vi "Feeding.vi"(8 "error In":errorcluster) -> (0 "error out":errorcluster)   [LabVIEW 2017]
uses:
  Controls/LOADING_DISPLAY.ctl
  <vilib>/Utility/error.llb/DialogType.ctl
  Controls/Feed_Cyc_Data.ctl
  Controls/QUEUE_STATES.ctl
  Controls/Feed_St.ctl
  <vilib>/Utility/file.llb/Read Delimited Spreadsheet (string).vi
  <vilib>/Instr/_visa.llb/VISA Configure Serial Port (Instr).vi
panel:
  out "logical AND":bool
  out "element":u16
  out "Boolean array":bool[](array[boolean])
  out "output cluster 2":cluster{"RECIPE INDEX":i32, "COMBI BIN":i32}
  in  "Close _Door":bool
  out "raw scan code":string
  in  "BYPASS SCN":bool
  in  "String":string
  out "Scanner Comm":bool
  out "Stop scanner":bool
  out "CYCLE STATUS":string
  out "CURRENT PLAN":T1
  out "SCAN CODE:":string
  out "Selected Plan structure":string[][](table)
  out "Plan Selected:":string
  out "USER:-":string
  in  "Stop":bool
  out "DATE/TIME":string
  out "Screen Name":string
  # "DOOR NUMBER"
  # "SCANNED CODE"
  # "FEEDER STATUS"
  # "DOOR NUMBER"
  # "SCANNED CODE"
  # "FEEDER STATUS"
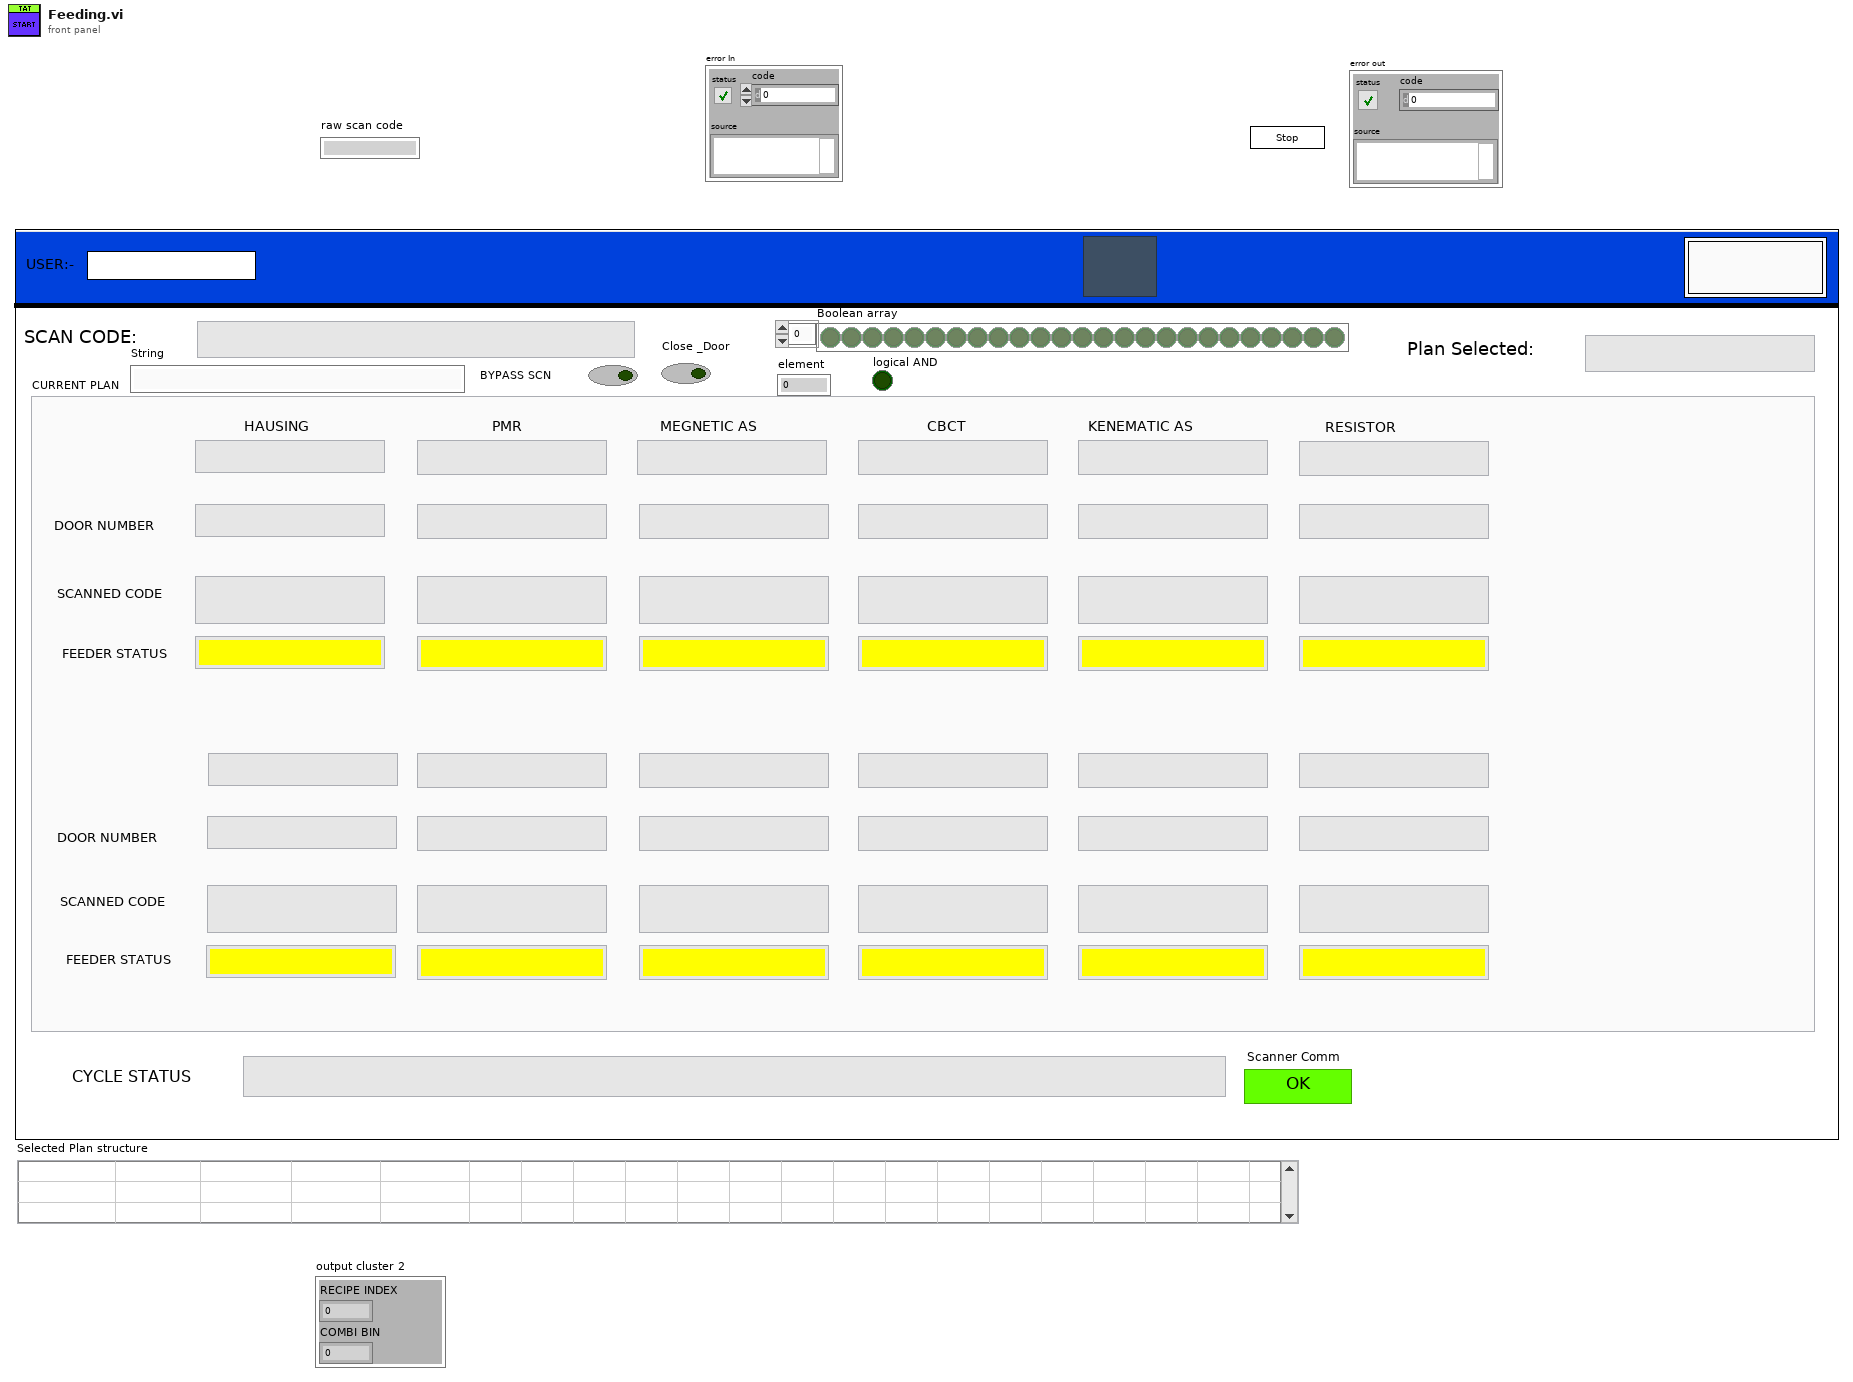
[diagram p1: front panel]
types:
  T1 = typedef "LOADING_DISPLAY.ctl" = cluster{"HAUSING":string, "PMR":string, "MEGNETIC AS":string, "CBCT":string, "KENEMATIC AS":string, "RESISTOR":string, "HAUSING DOOR":string, "PMR DOOR":string, "MAGNETIC AS DOOR":string, "CBCT DOOR":string, "KINEMATIC AS DOOR":string, "RESISTOR DOOR":string, "HAUSING SCAN QR":string, "PMR SCAN QR":string, "MAGNETIC SCAN QR":string, "CBCT SCAN QR":string, "KINEMATIC SCAN QR":string, "RESISTOR SCAN QR":string, "HAUSING FEED STATUS":string, "PMR FEED STATUS":string, "MAGNETIC AS FEEED STATUS":string, "CBCT FEED STATUS":string, "KINEMATIC AS FEED STATUS":string, "RESISTOR 1 FEED STATUS":string, "HAUSING 2":string, "PMR 2":string, "MEGNETIC AS 2":string, "CBCT 2":string, "KENEMATIC AS 2":string, "RESISTOR 2":string, "HAUSING DOOR 4":string, "PMR DOOR 4":string, "MAGNETIC AS DOOR 4":string, "CBCT DOOR 4":string, "KINEMATIC AS DOOR 4":string, "RESISTOR 1 DOOR 4":string, "HAUSING 2 SCAN QR":string, "PMR 2 SCAN QR":string, "MAGNETIC 2 SCAN QR":string, "CBCT 2 SCAN QR":string, "KINEMATIC 2 SCAN QR":string, "RESISTOR 2 SCAN QR":string, "HAUSING FEED STATUS 2":string, "PMR FEED STATUS 2":string, "MAGNETIC AS FEEED STATUS 2":string, "CBCT FEED STATUS 2":string, "KINEMATIC AS FEED STATUS 2":string, "RESISTOR 1 FEED STATUS 2":string}
  T2 = typedef "Feed_Cyc_Data.ctl" = cluster{"Cycle_Plan":path, "Plan_Data":string[][], "Scanned_Data":string[], "Scanned Chld Part":cluster{"Selected Door No":string, "child part code":string, "chld prt Row":i32, "Chld Prt Index":i32, "Scanned Data":string}, "feed Status Indi":refnum<vi>[], "Recipe Selected":cluster{"Bin/Box Mode":i32, "Selected Section":i32, "SELTED RECP & COMBI BIN":cluster{i32, i32}, "SELECTED RECIPE":string}}
  T3 = typedef "DialogType.ctl" = u16
  T4 = enum32{"invalid app kind", "Development System", "Run Time System", "Student Edition", "Embedded LabVIEW", "Evaluation", "Custom"}
  T5 = typedef "QUEUE_STATES.ctl" = enum16{"CREATE Q", "EN Q", "DE Q", "CLOSE Q"}
  T6 = cluster{"Printer IP":string, "PLC IP Address":string, "Scanner Com":refnum<visa-resource-name>}
  T7 = typedef "Feed_St.ctl" = enum16{"Int 2", "Cluster_update", "Read_Plan", "QR_Scanned", "Int", "SaveReport ", "Error_Handler", "Wait", "Close_Door", "Stop"}
  T8 = cluster{"Selected Door No":string, "child part code":string, "chld prt Row":i32, "Chld Prt Index":i32, "Scanned Data":string}
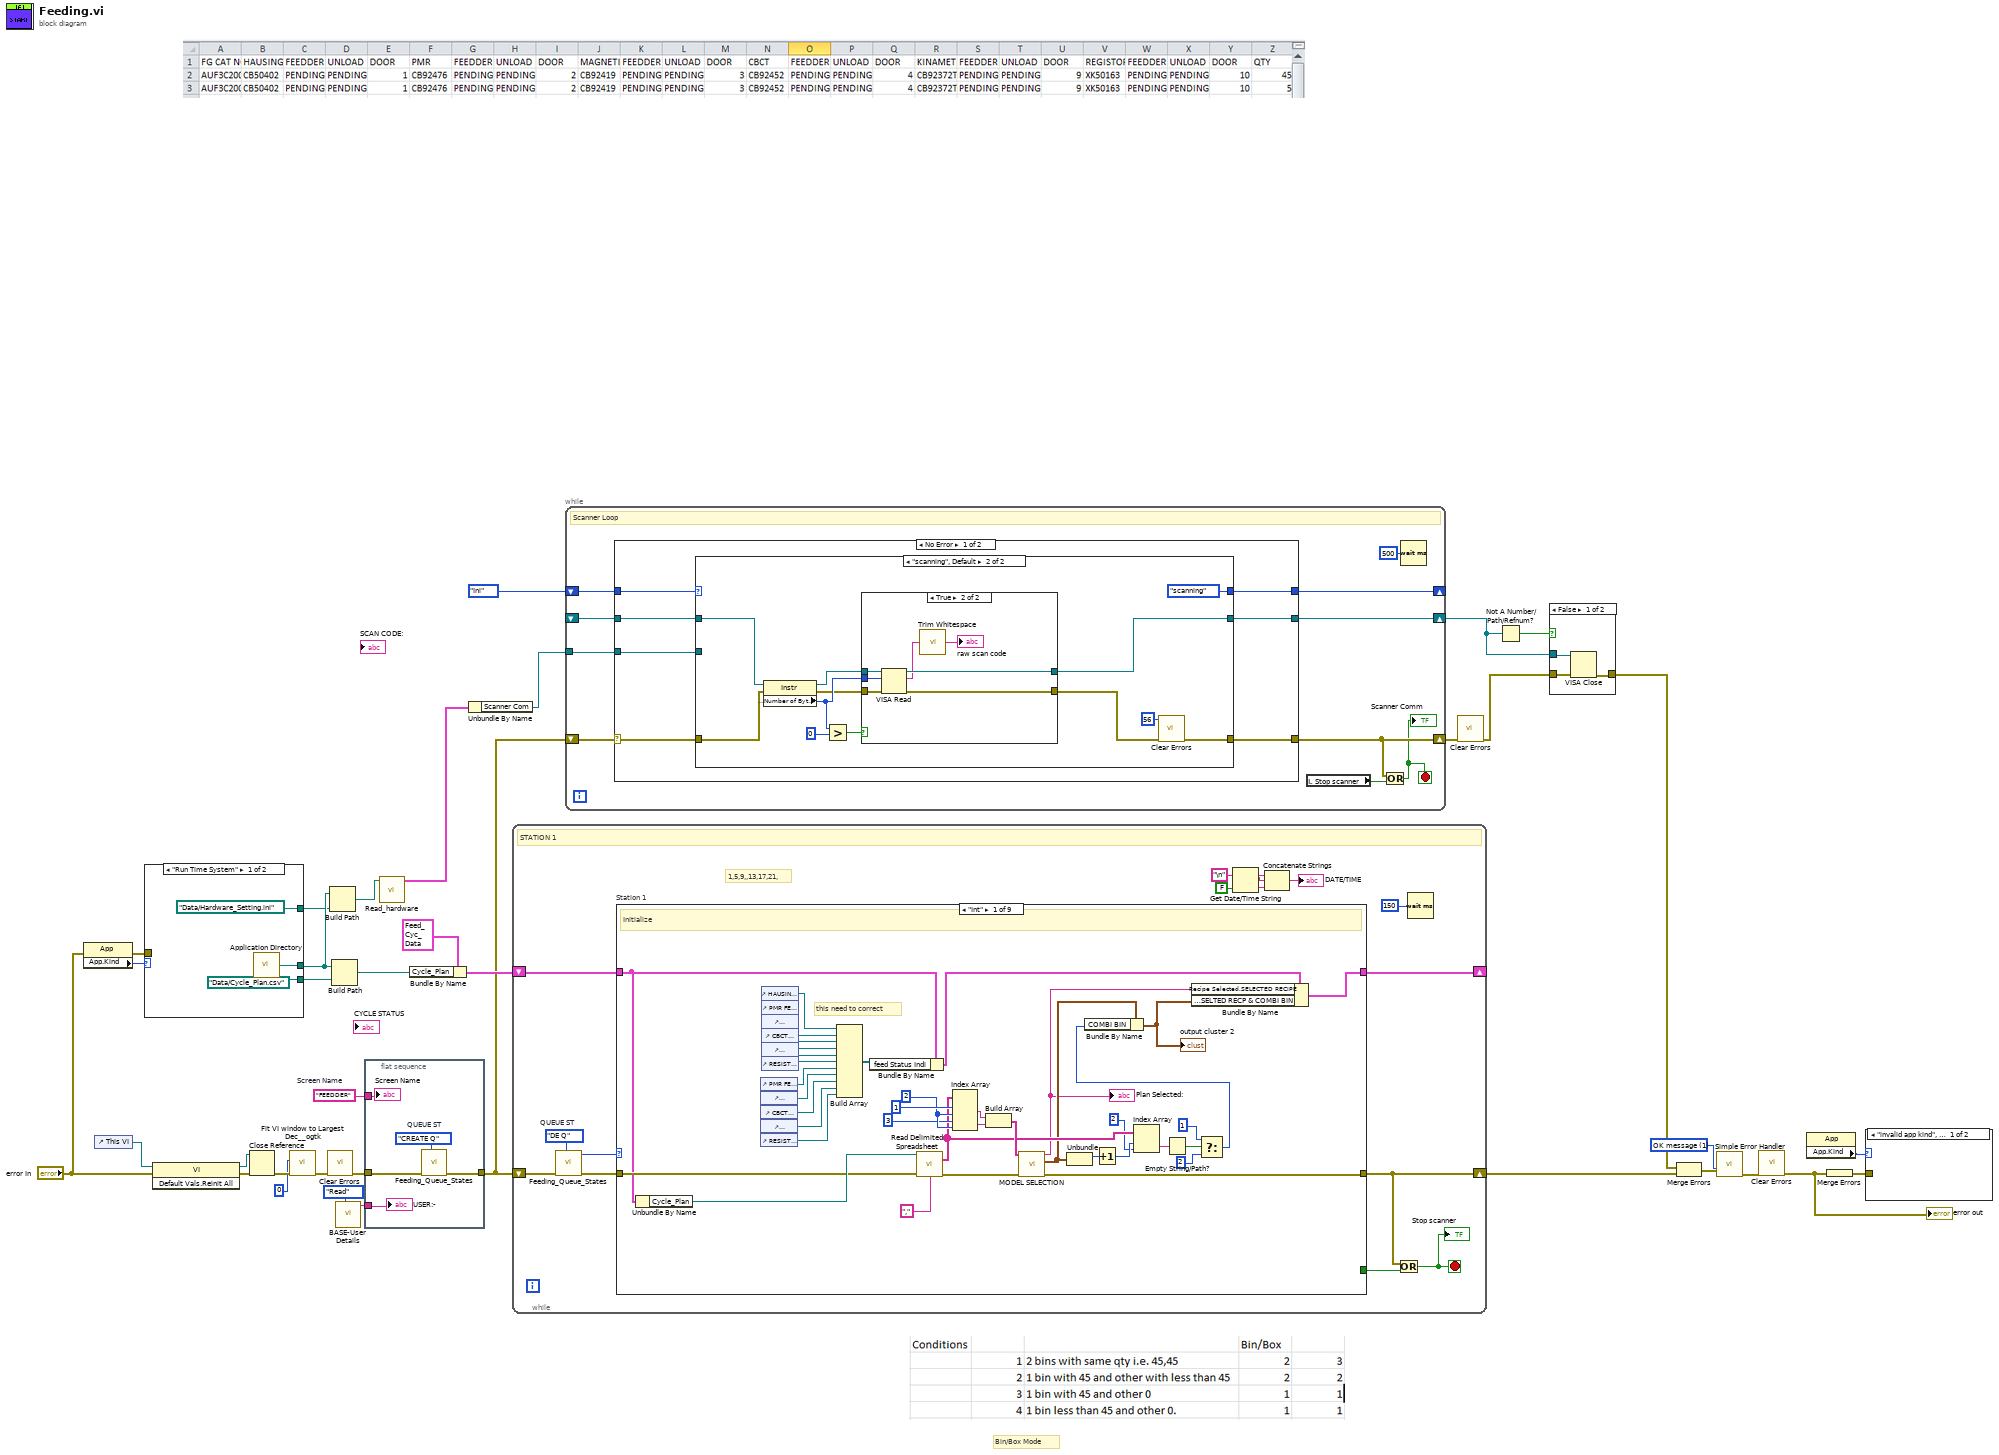
[diagram p0: block diagram]
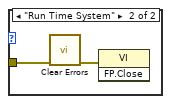
[diagram p2: hidden frame]
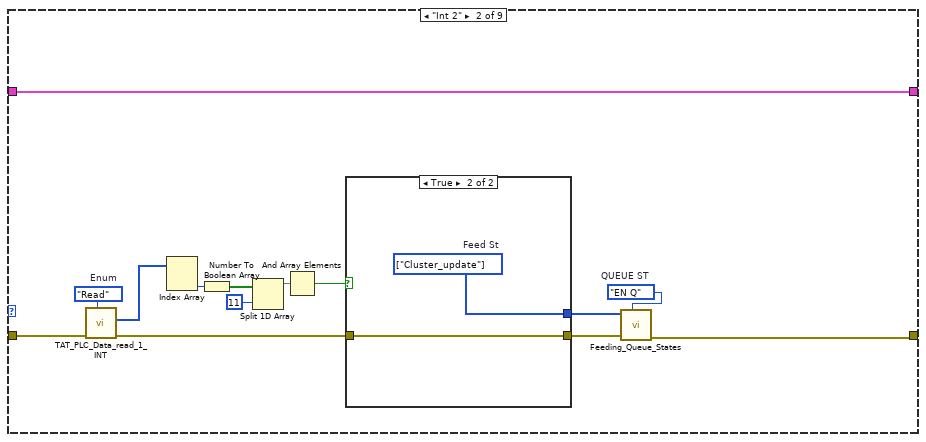
[diagram p3: hidden frame]
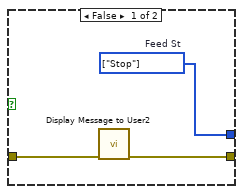
[diagram p4: hidden frame]
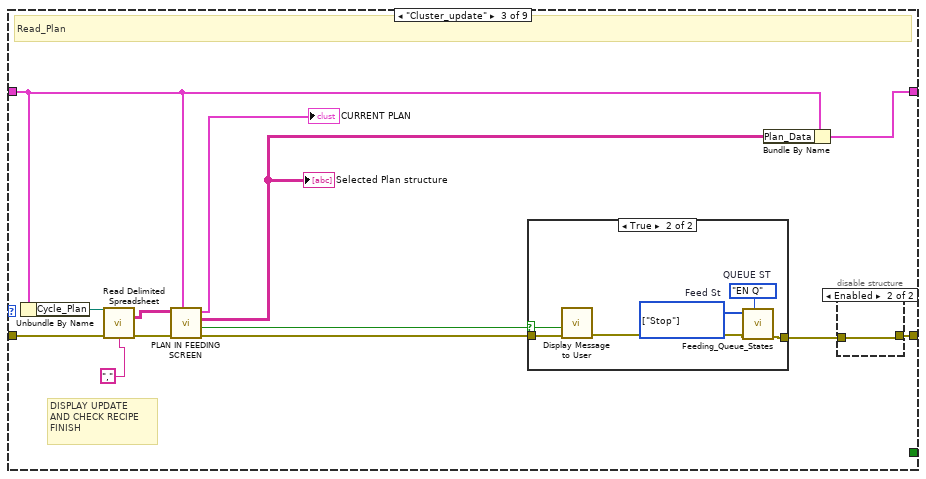
[diagram p5: hidden frame]
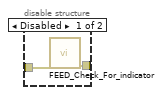
[diagram p6: hidden frame]
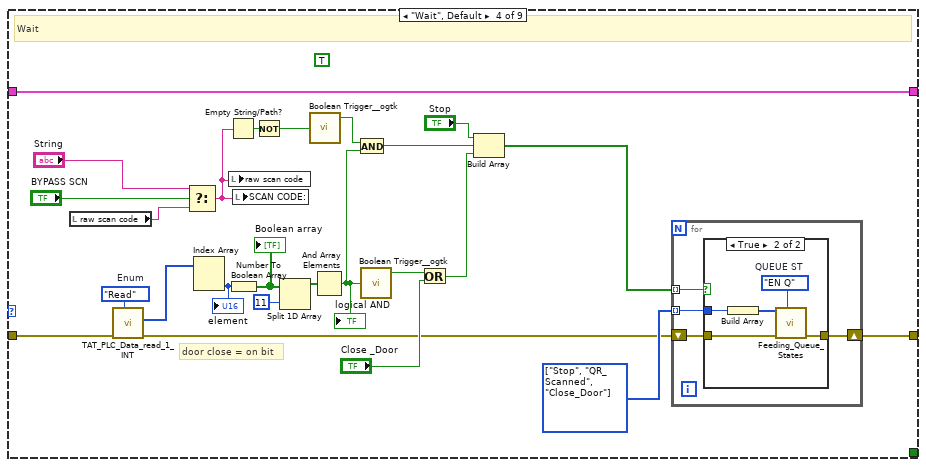
[diagram p8: hidden frame]
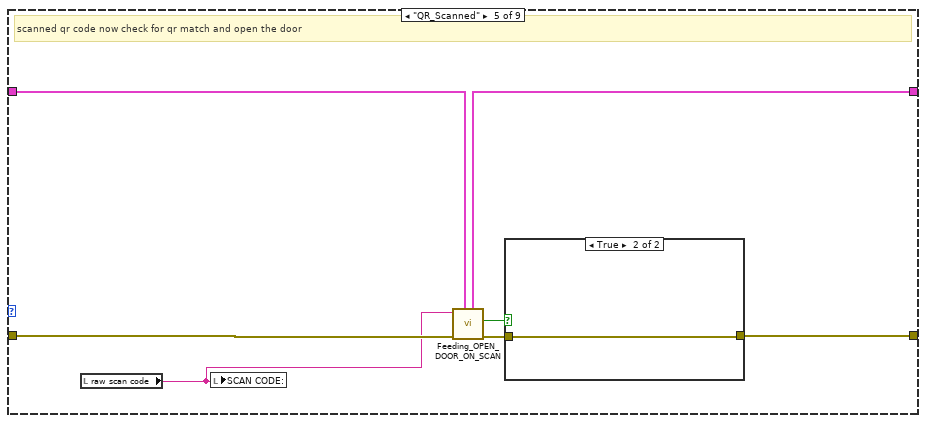
[diagram p10: hidden frame]
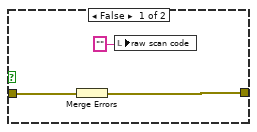
[diagram p11: hidden frame]
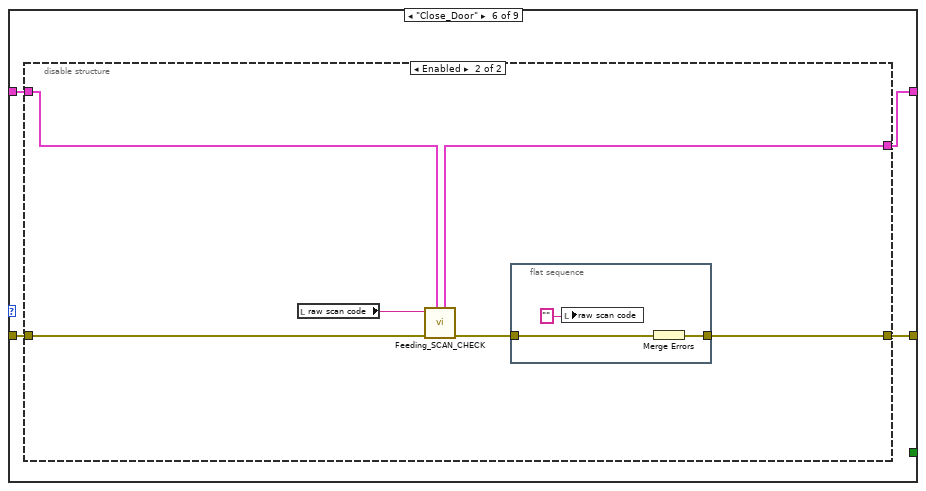
[diagram p12: hidden frame]
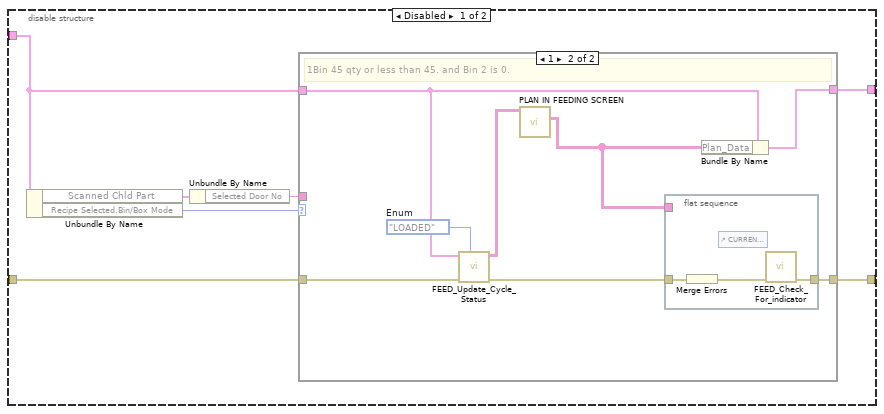
[diagram p13: hidden frame]
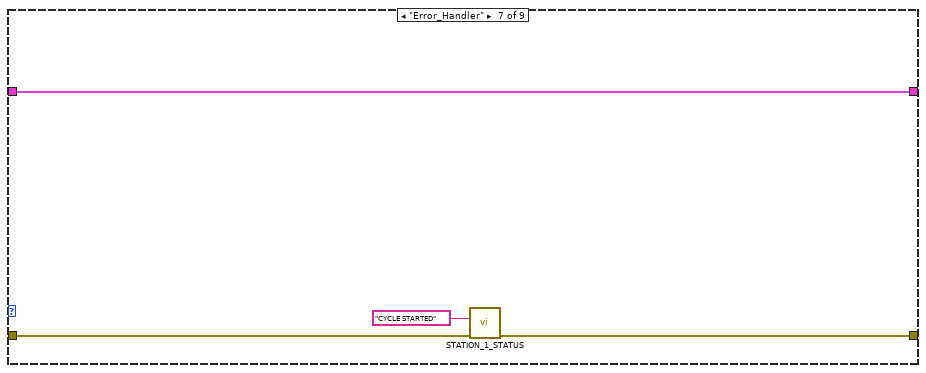
[diagram p15: hidden frame]
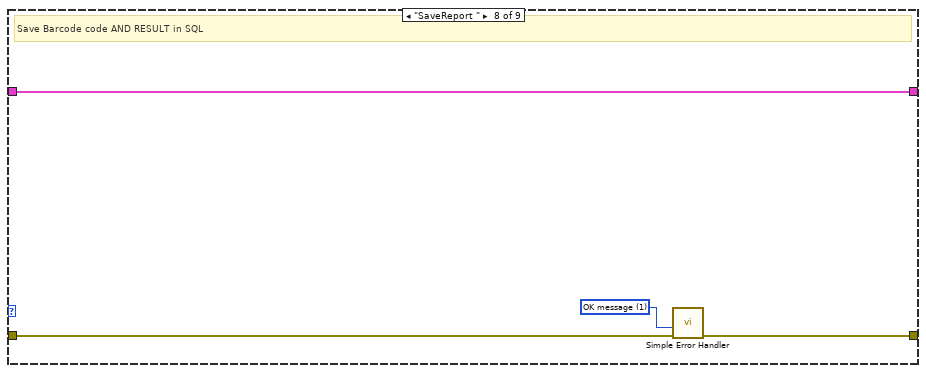
[diagram p16: hidden frame]
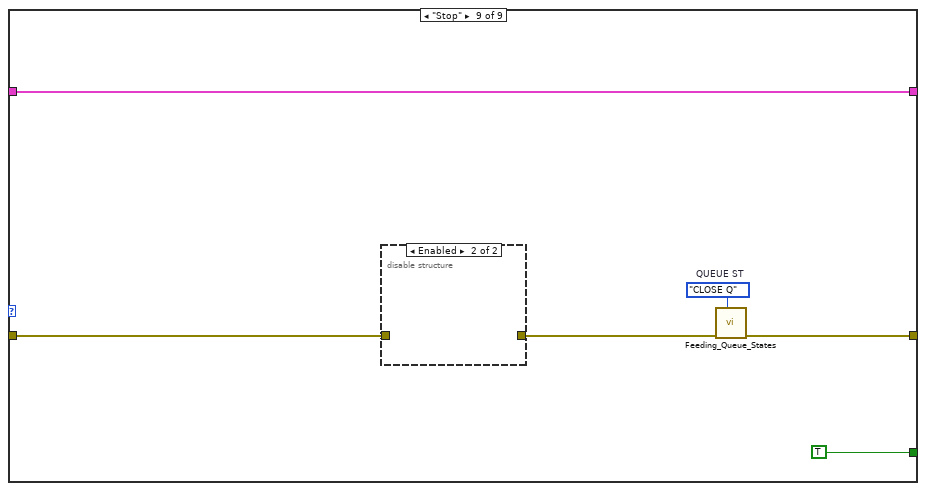
[diagram p17: hidden frame]
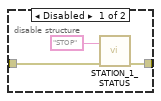
[diagram p18: hidden frame]
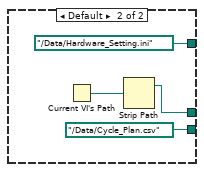
[diagram p19: hidden frame]
diagram:
  w17 = "FEEDDER"  # Screen Name
  w29 = T3 1 items=["no dialog", "OK message", "continue or stop message", "OK message + warnings", "continue/stop + warnings"] ("type of dialog (OK msg:1)")
  # "Bin/Box Mode"
  n1 = property class="App"(error in="error In") -> (error out=w25:errorcluster, "App.Kind"=w27:T4)  [unwired: 1 in, 1 out]
  n2 = control-ref of="This VI"() -> (w36:refnum<vi>)
  n3 = case shown="\"Run Time System\"" w27 {
    tunnel: [path "Data/Cycle_Plan.csv" ("path") path "../Data/Cycle_Plan.csv" ("path")] -> w26
    tunnel: [w37 w41] -> w6
    tunnel: w25 -> [_ _]
    tunnel: [path "Data/Hardware_Setting.ini" ("path") path "../Data/Hardware_Setting.ini" ("path")] -> w5
    frame "Run Time System" {
      n4 = call <vilib>:"Application Directory.vi"() -> ("Application Directory"=w37:path)
    }
    frame Default {
      n5 = Current VI's Path() -> (path=w42:path)
      n6 = Strip Path(path=w42) -> (stripped path=w41:path)  [unwired: 1 out]
    }
  }
  n7 = invoke class="VI" method="Default Vals.Reinit All"(reference=w36, error in="error In") -> (reference out=w34:refnum<vi>, error out=w35:errorcluster)  [unwired: 1 in, 1 out]
  n8 = Close Reference(reference=w34, error in (no error)=w35) -> (error out=w33:errorcluster)
  n9 = call <userlib>:"Fit VI window to Largest Dec__ogtk.vi"("error in (no error)"=w33, "border spacing (2 px)"=0) -> ("error out"=w23:errorcluster)  [unwired: 4 in, 1 out]
  n10 = call <vilib>:"Clear Errors.vi"("error in (no error)"=w23) -> ("error out"=w10:errorcluster)  [unwired: 5 in, 1 out]
  n11 = Build Path(base path=w6, name or relative path=w5) -> (appended path=w4:path)
  n12 = Build Path(base path=w6, name or relative path=w26) -> (appended path=w19:path)
  n13 = call "BASE-User Details.vi"("Enum"=enum16{"Read", "Write"}."Read") -> ("User Name Out"=w30:string)  [unwired: 9 in, 1 out]
  n14 = flat-sequence {
    tunnel: [w45] -> w11
    tunnel: w10 -> [w46]
    tunnel: w30 -> [w48]
    tunnel: w17 -> [w47]
    frame #0 {
      w44 = QUEUE_STATES."CREATE Q"  # QUEUE ST
      n15 = call "Feeding_Queue_States.vi"("QUEUE ST"=w44, "error in"=w46) -> ("error OUT"=w45:errorcluster)  [unwired: 8 in, 1 out]
      "USER:-" <- w48
      "Screen Name" <- w47
    }
  }
  n16 = call "Read_hardware.vi"("configuration file path"=w4) -> ("data"=w8:T6)  [unwired: 10 in]
  n17 = Bundle By Name(cluster=T2 {"Cycle_Plan"=path "", "Plan_Data"=[], "Scanned_Data"=[], "Scanned Chld Part"={"Selected Door No"="", "child part code"="", "chld prt Row"=0, "Chld Prt Index"=0, "Scanned Data"=""}, "feed Status Indi"=[], "Recipe Selected"={"Bin/Box Mode"=0, "Selected Section"=0, "SELTED RECP & COMBI BIN"={0, 0}, "SELECTED RECIPE"=""}}, "Cycle_Plan"=w19) -> (w18:T2)
  n18 = Unbundle By Name(w8) -> ("Scanner Com"=w7:refnum<visa-resource-name>)
  n19 = while {
    shift-right: [w55] -> _
    shift-left: w18 -> [w56]
    shift-right: [w53] -> w9
    shift-left: w11 -> [w52]
    stop <- w54 stop-if-true
    w50 = QUEUE_STATES."DE Q"  # QUEUE ST
    # "1,5,9,,13,17,21,"
    # "STATION 1"
    n20 = call "Feeding_Queue_States.vi"("QUEUE ST"=w50, "error in"=w52) -> ("error OUT"=w51:errorcluster, "Feed ST"=w49:T7)  [unwired: 8 in]
    n21 = case "Station 1" shown="\"Int\"" w49 {
      tunnel: [_ _ _ _ _ _ _ _ TRUE] -> w57
      tunnel: [w64 w104 w127 w165 w180 w192 w224 w229 w231] -> w53
      tunnel: w51 -> [w86 w108 w132 w154 w185 w193 w225 w228 w235]
      tunnel: w56 -> [w77 w115 w122 w168 w182 w191 w223 w227 w234]
      tunnel: [w78 w115 w126 w168 w181 w190 w223 w227 w234] -> w55
      frame "Int" {
        w83 = 2
        # "this need to correct"
        # "Initialize"
        n22 = Unbundle By Name(w77) -> ("Cycle_Plan"=w89:path)
        n23 = control-ref of="PMR FEED STATUS 2"() -> (w97:refnum<vi>)
        n24 = control-ref of="MAGNETIC AS FEEED STATUS 2"() -> (w98:refnum<vi>)
        n25 = control-ref of="CBCT FEED STATUS 2"() -> (w99:refnum<vi>)
        n26 = control-ref of="KINEMATIC AS FEED STATUS 2"() -> (w100:refnum<vi>)
        n27 = control-ref of="RESISTOR 1 FEED STATUS 2"() -> (w101:refnum<vi>)
        n28 = control-ref of="HAUSING FEED STATUS"() -> (w91:refnum<vi>)
        n29 = control-ref of="PMR FEED STATUS"() -> (w92:refnum<vi>)
        n30 = control-ref of="MAGNETIC AS FEEED STATUS"() -> (w93:refnum<vi>)
        n31 = control-ref of="CBCT FEED STATUS"() -> (w94:refnum<vi>)
        n32 = control-ref of="KINEMATIC AS FEED STATUS"() -> (w95:refnum<vi>)
        n33 = control-ref of="RESISTOR 1 FEED STATUS"() -> (w96:refnum<vi>)
        n34 = Build Array(w91, w92, w93, w94, w95, w96, w97, w98, w99, w100, w101) -> (w90:refnum<vi>[])
        n35 = Bundle By Name(cluster=w77, "feed Status Indi"=w90) -> (w79:T2)
        n36 = call-poly <vilib>:"Read Delimited Spreadsheet.vi"("file path (dialog if empty)"=w89, "error in (no error)"=w86, "delimiter (\\t)"=",") -> ("all rows"=w76:string[][], "error out"=w85:errorcluster)  [unwired: 7 in, 4 out]
        n37 = Index Array(array=w76, index (row) #1=1, index (col) #1=w83, index (row) #2=3, index (col) #2=w83) -> (element #1=w81:string, element #2=w80:string)
        n38 = Build Array(w81, w80) -> (w88:string[])
        n39 = call "MODEL SELECTION.vi"("error in (no error)"=w85, "Plan List"=w88) -> ("error out 2"=w64:errorcluster, "SELECTED RECIPE\nand COMBI OF BIN- INDEX"=w68:cluster{"RECIPE INDEX":i32, "COMBI BIN":i32}, "Plan Selected"=w65:string)  [unwired: 7 in]
        "Plan Selected:" <- w65
        n40 = Unbundle(w68) -> ("RECIPE INDEX"=w75:i32)  [unwired: 1 out]
        n41 = Increment(x=w75) -> (x+1=w74:i32)
        n42 = Index Array(array=w76, index (row)=w74, index (col)=2) -> (element=w72:string)
        n43 = Empty String/Path?(string/path=w72) -> (empty?=w71:bool)
        n44 = Select(t=1, s=w71, f=2) -> (s? t:f=w66:i32)
        n45 = Bundle By Name(cluster=w68, "COMBI BIN"=w66) -> (w67:cluster{"RECIPE INDEX":i32, "COMBI BIN":i32})
        "output cluster 2" <- w67
        n46 = Bundle By Name(cluster=w79, "Recipe Selected.SELECTED RECIPE"=w65, "Recipe Selected.SELTED RECP & COMBI BIN"=w67) -> (w78:T2)
      }
      frame "Int 2" {
        w106 = QUEUE_STATES."EN Q"  # QUEUE ST
        w114 = enum16{"Read", "Write"}."Read"  # Enum
        n47 = call "TAT_PLC_Data_read_1_INT.vi"("Enum"=w114, "error in (no error)"=w108) -> ("error out"=w107:errorcluster, "Array 2"=w113:u16[])  [unwired: 8 in]
        n48 = Index Array(array=w113) -> (element #2=w112:u16)  [unwired: 2 in, 1 out]
        n49 = Number To Boolean Array(number=w112) -> (Boolean array=w111:bool[])
        n50 = Split 1D Array(array=w111, index=11) -> (first subarray=w109:bool[])  [unwired: 1 out]
        n51 = And Array Elements(Boolean array=w109) -> (logical AND=w102:bool)
        n52 = case shown="True" w102 {
          tunnel: w107 -> [w117 w119]
          tunnel: [w116 w119] -> w103
          tunnel: [w118 w120] -> w105
          frame False {
            w118 = T7[] [enum."Stop"] items=["Int 2", "Cluster_update", "Read_Plan", "QR_Scanned", "Int", "SaveReport ", "Error_Handler", "Wait", "Close_Door", "Stop"]  # Feed St
            n53 = call "Display Message to User2"("error in (no error)"=w117) -> ("error out"=w116:errorcluster)  [unwired: 9 in, 1 out]
          }
          frame True {
            w120 = T7[] [enum."Cluster_update"] items=["Int 2", "Cluster_update", "Read_Plan", "QR_Scanned", "Int", "SaveReport ", "Error_Handler", "Wait", "Close_Door", "Stop"]  # Feed St
          }
        }
        n54 = call "Feeding_Queue_States.vi"("QUEUE ST"=w106, "error in"=w103, "Feed St"=w105) -> ("error OUT"=w104:errorcluster)  [unwired: 7 in, 1 out]
      }
      frame "Cluster_update" {
        # "DISPLAY UPDATE\nAND CHECK RECIPE\nFINISH"
        # "Read_Plan"
        n55 = Unbundle By Name(w122) -> ("Cycle_Plan"=w131:path)
        n56 = call-poly <vilib>:"Read Delimited Spreadsheet.vi"("file path (dialog if empty)"=w131, "error in (no error)"=w132, "delimiter (\\t)"=",") -> ("all rows"=w129:string[][], "error out"=w124:errorcluster)  [unwired: 7 in, 4 out]
        n57 = call "PLAN IN FEEDING SCREEN.vi"("LOOP DATA IN"=w122, "error IN"=w124, "PLAN In"=w129) -> ("error out"=w125:errorcluster, "NO EMPTY CMPLT?"=w121:bool, "PLAN Out"=w130:string[][], "CURRENT PLAN"=→"CURRENT PLAN":T1)  [unwired: 4 in]
        "Selected Plan structure" <- w130
        n58 = case shown="True" w121 {
          selector: w121 -> [_ w138]
          tunnel: w125 -> [w137 w140]
          tunnel: [w137 w142] -> w128
          frame False {
          }
          frame True {
            w141 = T7[] [enum."Stop"] items=["Int 2", "Cluster_update", "Read_Plan", "QR_Scanned", "Int", "SaveReport ", "Error_Handler", "Wait", "Close_Door", "Stop"]  # Feed St
            w143 = QUEUE_STATES."EN Q"  # QUEUE ST
            n59 = call "Display Message to User"("error in (no error)"=w140, "Enable"=w138) -> ("error out"=w139:errorcluster)  [unwired: 8 in, 1 out]
            n60 = call "Feeding_Queue_States.vi"("QUEUE ST"=w143, "error in"=w139, "Feed St"=w141) -> ("error OUT"=w142:errorcluster)  [unwired: 7 in, 1 out]
          }
        }
        n61 = Bundle By Name(cluster=w122, "Plan_Data"=w130) -> (w126:T2)
        n62 = disable-structure shown="Enabled" {
          disable-tunnel: w128 -> [w135 w136]
          disable-tunnel: [w134 w136] -> w127
          frame Disabled {
            n63 = call "FEED_Check_For_indicator.vi"("error in (no error)"=w135) -> ("error out"=w134:errorcluster)  [unwired: 10 in]
          }
          frame Enabled {
          }
        }
      }
      frame "Wait", Default {
        (unwired) TRUE
        w152 = enum16{"Read", "Write"}."Read"  # Enum
        w161 = T7[] [enum."Stop", enum."QR_Scanned", enum."Close_Door"] items=["Int 2", "Cluster_update", "Read_Plan", "QR_Scanned", "Int", "SaveReport ", "Error_Handler", "Wait", "Close_Door", "Stop"] ("Array")
        # "door close = on bit"
        # "Wait"
        n64 = local read "raw scan code"() -> (w160:string)
        n65 = call "TAT_PLC_Data_read_1_INT.vi"("Enum"=w152, "error in (no error)"=w154) -> ("error out"=w153:errorcluster, "Array 2"=w151:u16[])  [unwired: 8 in]
        n66 = Select(t="String", s="BYPASS SCN", f=w160) -> (s? t:f=w157:string)
        n67 = Index Array(array=w151) -> (element #2=w148:u16)  [unwired: 2 in, 1 out]
        "element" <- w148
        n68 = Empty String/Path?(string/path=w157) -> (empty?=w164:bool)
        n69 = local write "raw scan code"(w157) -> ()
        n70 = Number To Boolean Array(number=w148) -> (Boolean array=w147:bool[])
        "Boolean array" <- w147
        n71 = local write "SCAN CODE:"(w157) -> ()
        n72 = Not(x=w164) -> (.not. x?=w156:bool)
        n73 = Split 1D Array(array=w147, index=11) -> (first subarray=w145:bool[])  [unwired: 1 out]
        n74 = call <userlib>:"Boolean Trigger__ogtk.vi"("Boolean Input"=w156) -> ("Rising Edge"=w155:bool)  [unwired: 1 in, 1 out]
        n75 = And Array Elements(Boolean array=w145) -> (logical AND=w144:bool)
        "logical AND" <- w144
        n76 = And(x=w155, y=w144) -> (x .and. y?=w150:bool)
        n77 = call <userlib>:"Boolean Trigger__ogtk.vi"("Boolean Input"=w144) -> ("Rising Edge"=w149:bool)  [unwired: 1 in, 1 out]
        n78 = Or(x=w149, y="Close _Door") -> (x .or. y?=w158:bool)
        n79 = Build Array("Stop", w150, w158) -> (w162:bool[])
        n80 = for {
          shift-right: [w171] -> w165
          shift-left: w153 -> [w172]
          tunnel: w162 -> [w170] mode=indexing
          tunnel: w161 -> [w169] mode=indexing
          n81 = case shown="True" w170 {
            tunnel: w172 -> [w173 w177]
            tunnel: [w173 w176] -> w171
            tunnel: w169 -> [_ w175]
            frame False {
            }
            frame True {
              w178 = QUEUE_STATES."EN Q"  # QUEUE ST
              n82 = Build Array(w175) -> (w174:T7[])
              n83 = call "Feeding_Queue_States.vi"("QUEUE ST"=w178, "error in"=w177, "Feed St"=w174) -> ("error OUT"=w176:errorcluster)  [unwired: 7 in, 1 out]
            }
          }
        }
      }
      frame "QR_Scanned" {
        # "scanned qr code now check for qr match and open the door"
        n84 = local read "raw scan code"() -> (w183:string)
        n85 = local write "SCAN CODE:"(w183) -> ()
        n86 = call "Feeding_OPEN_DOOR_ON_SCAN.vi"("CYCLE DATA IN"=w182, "error in (no error)"=w185, "raw scan code"=w183) -> ("error out"=w184:errorcluster, "search valid ?"=w179:bool, "CYCLE DATA OUT"=w181:T2)  [unwired: 6 in]
        n87 = case shown="True" w179 {
          tunnel: w184 -> [w188 w189]
          tunnel: [w187 w189] -> w180
          frame False {
            n88 = Merge Errors(w188) -> (w187:errorcluster)
            n89 = local write "raw scan code"("") -> ()
          }
          frame True {
          }
        }
      }
      frame "Close_Door" {
        n90 = disable-structure shown="Enabled" {
          disable-tunnel: w193 -> [w200 w219]
          disable-tunnel: [w199 w214] -> w192
          disable-tunnel: w191 -> [w196 w217]
          disable-tunnel: [w195 w216] -> w190
          frame Disabled {
            n91 = Unbundle By Name(w196) -> ("Scanned Chld Part"=w197:T8, "Recipe Selected.Bin/Box Mode"=w194:i32)
            n92 = Unbundle By Name(w197) -> ("Selected Door No"=w198:string)
            n93 = case shown="1" w194 {
              tunnel: w200 -> [w201 w209]
              tunnel: [w201 w204] -> w199
              tunnel: w198 -> [_ _]
              tunnel: w196 -> [w202 w206]
              tunnel: [w202 w210] -> w195
              frame 0, Default {
              }
              frame 1 {
                w207 = enum16{"FEED", "LOADED"}."LOADED"  # Enum
                # "1Bin 45 qty or less than 45. and Bin 2 is 0."
                n94 = call "FEED_Update_Cycle_Status.vi"("Enum"=w207, "error in (no error)"=w209, 11:w206) -> ("error out"=w208:errorcluster, "output array"=w205:string[][])  [unwired: 6 in, 1 out]
                n95 = call "PLAN IN FEEDING SCREEN.vi"("PLAN In"=w205) -> ("PLAN Out"=w203:string[][])  [unwired: 6 in, 3 out]
                n96 = flat-sequence {
                  tunnel: w208 -> [w213]
                  tunnel: [w211] -> w204
                  tunnel: w203 -> [_]
                  frame #0 {
                    n97 = Merge Errors(w213) -> (w212:errorcluster)
                    n98 = control-ref of="CURRENT PLAN"() -> ()  [unwired: 1 out]
                    n99 = call "FEED_Check_For_indicator.vi"("error in (no error)"=w212) -> ("error out"=w211:errorcluster)  [unwired: 10 in]
                  }
                }
                n100 = Bundle By Name(cluster=w206, "Plan_Data"=w203) -> (w210:T2)
              }
            }
          }
          frame Enabled {
            n101 = local read "raw scan code"() -> (w215:string)
            n102 = call "Feeding_SCAN_CHECK.vi"("CYCLE DATA IN"=w217, "error in (no error)"=w219, "raw scan code"=w215) -> ("error out"=w218:errorcluster, "CYCLE DATA OUT"=w216:T2)  [unwired: 7 in]
            n103 = flat-sequence {
              tunnel: w218 -> [w222]
              tunnel: [w220] -> w214
              frame #0 {
                n104 = local write "raw scan code"("") -> ()
                n105 = Merge Errors(w222) -> (w220:errorcluster)
              }
            }
          }
        }
      }
      frame "Error_Handler" {
        n106 = call "STATION_1_STATUS.vi"("error in (no error)"=w225, "STATUS"="CYCLE STARTED" ("Cycle Status")) -> ("error out"=w224:errorcluster)  [unwired: 9 in]
      }
      frame "SaveReport " {
        w230 = T3 1 items=["no dialog", "OK message", "continue or stop message", "OK message + warnings", "continue/stop + warnings"] ("type of dialog (OK msg:1)")
        # "Save Barcode code AND RESULT in SQL"
        n107 = call <vilib>:"Simple Error Handler.vi"("type of dialog (OK msg:1)"=w230, "error in (no error)"=w228) -> ("error out"=w229:errorcluster)  [unwired: 3 in, 4 out]
      }
      frame "Stop" {
        w233 = QUEUE_STATES."CLOSE Q"  # QUEUE ST
        n108 = disable-structure shown="Enabled" {
          disable-tunnel: w235 -> [w238 _]
          disable-tunnel: [w237 _] -> w232
          frame Disabled {
            n109 = call "STATION_1_STATUS.vi"("error in (no error)"=w238, "STATUS"="STOP" ("Cycle Status")) -> ("error out"=w237:errorcluster)  [unwired: 9 in]
          }
          frame Enabled {
          }
        }
        n110 = call "Feeding_Queue_States.vi"("QUEUE ST"=w233, "error in"=w232) -> ("error OUT"=w231:errorcluster)  [unwired: 8 in, 1 out]
      }
    }
    n111 = Get Date/Time String(want seconds? (F)=FALSE) -> (date string=w61:string, time string=w60:string)  [unwired: 2 in]
    n112 = Concatenate Strings(w61, "\n", w60) -> (→"DATE/TIME":string)
    n113 = Or(x=w53, y=w57) -> (x .or. y?=w54:bool)
    "Stop scanner" <- w54
    n114 = Wait (ms)(milliseconds to wait=u32 150) -> ()  [unwired: 1 out]
  }
  n115 = while {
    shift-right: [w248] -> w15
    shift-left: w11 -> [w249]
    shift-right: [w246] -> _
    shift-left: enum16{"Ini", "scanning", "Close"}."Ini" -> [w247]
    tunnel: w7 -> [w245]
    shift-right: [w244] -> w12
    shift-left: _ -> [w243]
    stop <- w242 stop-if-true
    # "Scanner Loop"
    n116 = case shown="No Error" w249 {
      selector: w249 -> [w256 w286]
      tunnel: [w255 w285] -> w248
      tunnel: w247 -> [w254 _]
      tunnel: [w253 enum16{"Ini", "scanning", "Close"}."scanning"] -> w246
      tunnel: w245 -> [w252 _]
      tunnel: [w251 w283] -> w244
      tunnel: w243 -> [w250 w283]
      frame No Error {
        n117 = case shown="\"scanning\", Default" w254 {
          tunnel: w256 -> [w260 w264]
          tunnel: [w259 w272] -> w255
          tunnel: [enum16{"Ini", "scanning", "Close"}."scanning" enum16{"Ini", "scanning", "Close"}."scanning"] -> w253
          tunnel: w252 -> [w258 _]
          tunnel: [w257 w262] -> w251
          tunnel: w250 -> [_ w265]
          frame "Ini" {
            n118 = call-poly "VISA Configure Serial Port"("VISA resource name"=w258, "error in (no error)"=w260) -> ("VISA resource name out"=w257:refnum<visa-resource-name>, "error out"=w259:errorcluster)  [unwired: 12 in]
          }
          frame "scanning", Default {
            n119 = property class="Instr"(reference=w265, error in=w264) -> (reference out=w267:refnum<visa-resource-name>, error out=w268:errorcluster, "Serial Settings:Number of Bytes at Serial Port"=w269:u32)
            n120 = Greater?(x=w269, y=u32 0) -> (0:w270:bool)
            n121 = case shown="True" w270 {
              tunnel: w267 -> [w275 w282]
              tunnel: w268 -> [w274 w281]
              tunnel: w269 -> [_ w280]
              tunnel: [w275 w279] -> w262
              tunnel: [w274 w277] -> w263
              frame False {
              }
              frame True {
                n122 = VISA Read(VISA resource name=w282, byte count=w280, error in (no error)=w281) -> (VISA resource name out=w279:refnum<visa-resource-name>, read buffer=w278:string, error out=w277:errorcluster)  [unwired: 1 out]
                n123 = call <vilib>:"Trim Whitespace.vi"("string"=w278) -> ("trimmed string"=→"raw scan code":string)  [unwired: 1 in]
              }
            }
            n124 = call <vilib>:"Clear Errors.vi"("error in (no error)"=w263, "specific error code to clear (0: all)"=56) -> ("error out"=w272:errorcluster)  [unwired: 4 in, 1 out]
          }
        }
      }
      frame Error {
        n125 = Unbundle By Name(w286) -> ("code"=w287:i32)
        n126 = case shown="1" w287 {
          tunnel: w286 -> [w291 w293]
          tunnel: [w289 w292] -> w285
          frame 0, Default {
            w288 = T3 2 items=["no dialog", "OK message", "continue or stop message", "OK message + warnings", "continue/stop + warnings"] ("type of dialog (OK msg:1)")
            n127 = call <vilib>:"Simple Error Handler.vi"("type of dialog (OK msg:1)"=w288, "error in (no error)"=w291) -> ("error out"=w290:errorcluster)  [unwired: 3 in, 4 out]
            n128 = call <vilib>:"Clear Errors.vi"("error in (no error)"=w290) -> ("error out"=w289:errorcluster)  [unwired: 5 in, 1 out]
          }
          frame 1 {
            w294 = "THIS ERROR OCCURED AS SCREEN 1 IS NOT CONNECTED OR OFF"  # source
            # "Monitor not present/Off/disconnected"
            n129 = Bundle By Name(cluster=w293, "source"=w294) -> (w292:errorcluster)
          }
        }
      }
    }
    n130 = local read "Stop scanner"() -> (w240:bool)
    n131 = Or(x=w248, y=w240) -> (x .or. y?=w242:bool)
    "Scanner Comm" <- w242
    n132 = Wait (ms)(milliseconds to wait=u32 500) -> ()  [unwired: 1 out]
  }
  n133 = call <vilib>:"Clear Errors.vi"("error in (no error)"=w15) -> ("error out"=w13:errorcluster)  [unwired: 5 in, 1 out]
  n134 = Not A Number/Path/Refnum?(number/path/refnum=w12) -> (NaN/Path/Refnum?=w14:bool)
  n135 = case shown="False" w14 {
    tunnel: w13 -> [w297 w298]
    tunnel: w12 -> [w295 _]
    tunnel: [w296 w298] -> w3
    frame False {
      n136 = VISA Close(VISA resource name=w295, error in (no error)=w297) -> (error out=w296:errorcluster)
    }
    frame True {
    }
  }
  n137 = Merge Errors(w3, w9) -> (w32:errorcluster)
  n138 = call <vilib>:"Simple Error Handler.vi"("type of dialog (OK msg:1)"=w29, "error in (no error)"=w32) -> ("error out"=w2:errorcluster)  [unwired: 3 in, 4 out]
  n139 = call <vilib>:"Clear Errors.vi"("error in (no error)"=w2) -> ("error out"=w1:errorcluster)  [unwired: 5 in, 1 out]
  "error out" <- w1
  n140 = property class="App"() -> ("App.Kind"=w28:T4)  [unwired: 2 in, 2 out]
  n141 = Merge Errors(w1) -> (w21:errorcluster)
  n142 = case shown="\"invalid app kind\", Default" w28 {
    tunnel: w21 -> [_ w300]
    frame "invalid app kind", Default {
    }
    frame "Run Time System" {
      n143 = call <vilib>:"Clear Errors.vi"("error in (no error)"=w300) -> ("error out"=w299:errorcluster)  [unwired: 5 in, 1 out]
      n144 = invoke class="VI" method="FP.Close"(error in=w299) -> ()  [unwired: 2 in, 3 out]
    }
  }
